vi "产生电压序列.vi"(1 "Delt":dbl, 2 "Min":dbl, 3 "Max":dbl) -> (0 "Array":dbl[](array[numeric]))   [LabVIEW 2018]
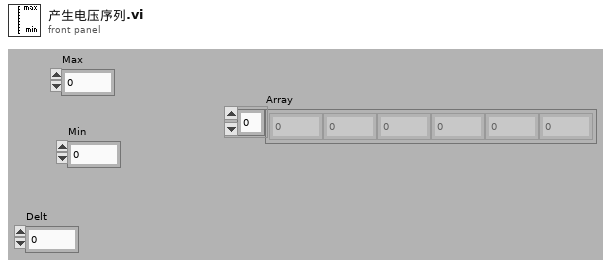
[diagram p1: front panel]
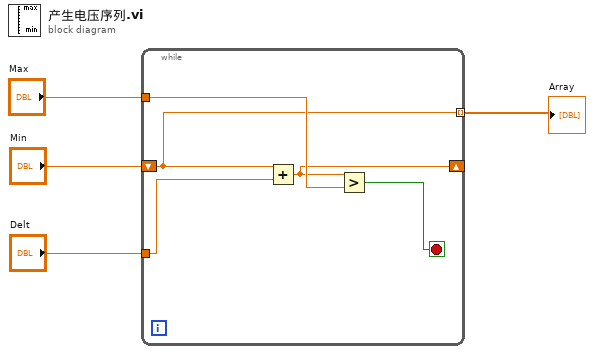
[diagram p0: block diagram]
diagram:
  n1 = while {
    tunnel: "Max" -> [w8]
    tunnel: "Delt" -> [w9]
    tunnel: [w5] -> w1 mode=indexing
    shift-right: [w6] -> _
    shift-left: "Min" -> [w5]
    stop <- w7 stop-if-true
    n2 = Add(x=w5, y=w9) -> (x+y=w6:dbl)
    n3 = Greater?(x=w6, y=w8) -> (0:w7:bool)
  }
  "Array" <- w1
